vi "LEER PUERTO SERIAL S FLOTANTE v2.vi"(4 "caracter terminador":string, 5 "read buffer":string, 6 "buffer de datos":dbl[](array[numeric]), 7 "buffer in":string) -> (0 "indicador de llegada de datos":bool, 2 "salida datos numericos":dbl[](array[numeric]), 3 "buffer out":string)   [LabVIEW 2017]
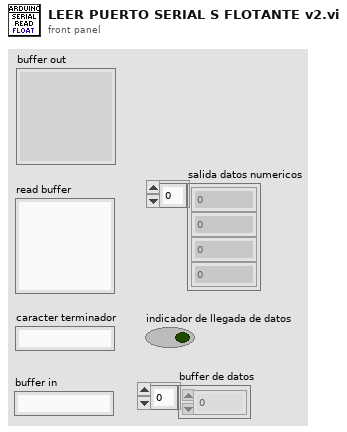
[diagram p1: front panel]
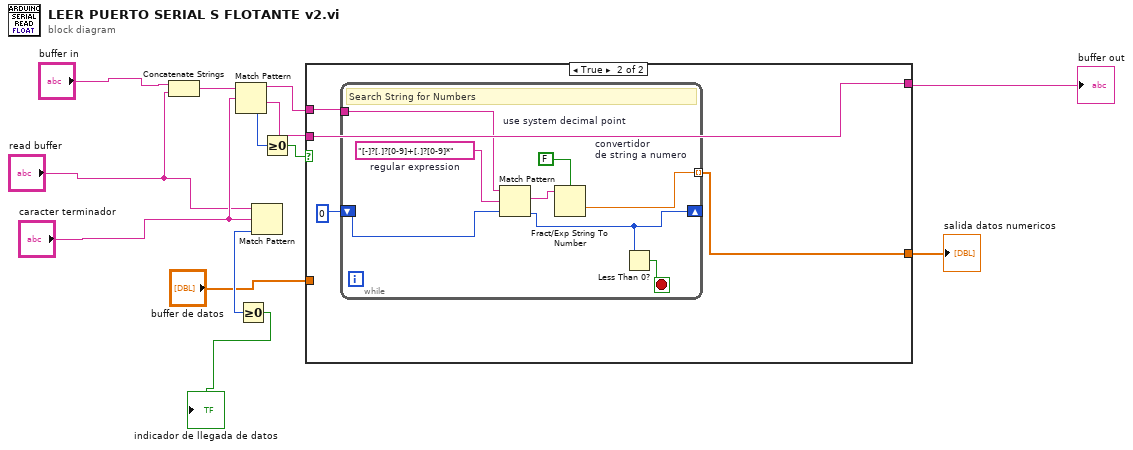
[diagram p0: block diagram]
diagram:
  n1 = Concatenate Strings("buffer in", "read buffer") -> (w6:string)
  n2 = Match Pattern(string=w6, regular expression="caracter terminador") -> (before substring=w5:string, after substring=w7:string, offset past match=w9:i32)  [unwired: 1 in, 1 out]
  n3 = Match Pattern(string="read buffer", regular expression="caracter terminador") -> (offset past match=w4:i32)  [unwired: 1 in, 3 out]
  n4 = Greater Or Equal To 0?(x=w4) -> (x >= 0?=→"indicador de llegada de datos":bool)
  n5 = Greater Or Equal To 0?(x=w9) -> (x >= 0?=w8:bool)
  n6 = case shown="True" w8 {
    tunnel: w7 -> [_ w19]
    tunnel: [w15 w19] -> w10
    tunnel: w5 -> [w15 w17]
    tunnel: [w14 w16] -> w2
    tunnel: "buffer de datos" -> [w14 _]
    frame False {
    }
    frame True {
      n7 = while {
        shift-left: 0 -> [w25]
        shift-right: [w22] -> _
        tunnel: [w27] -> w16 mode=indexing
        tunnel: w17 -> [w20]
        stop <- w26 stop-if-true
        w24 = FALSE  # use system decimal point
        w21 = "[-]?[.]?[0-9]+[.]?[0-9]*"  # regular expression
        # "Search String for Numbers"
        n8 = Match Pattern(string=w20, regular expression=w21, offset (0)=w25) -> (match substring=w23:string, offset past match=w22:i32)  [unwired: 2 out]
        n9 = Fract/Exp String To Number "convertidor\nde string a numero"(use system decimal point (T)=w24, string=w23) -> (number=w27:dbl)  [unwired: 2 in, 1 out]
        n10 = Less Than 0?(x=w22) -> (x < 0?=w26:bool)
      }
    }
  }
  "buffer out" <- w10
  "salida datos numericos" <- w2
